vi "ScaledWaveform-GetChannelsRefs.vi"(8 "Error in":errorcluster, 9 "Enabled?":bool, 11 "Device Ref in":T1 format="%.0x") -> (0 "Error out":errorcluster, 2 "Group Data Array":T2(array[cluster]) {"VS Refs" format="%.0x"}, 3 "Device Ref out":T1=18446744073709551615 format="%.0x")   [LabVIEW 2020, in "Waveform-Processing-Custom-Device Shared.lvlib" / "Scaled Waveform.lvlib"]
uses:
  Scaled Waveform.lvlib
  <vilib>/NI VeriStand/Custom Device API/Custom Device Item Ref.ctl
  Constants.vi
  <vilib>/NI VeriStand/Custom Device Tools/Custom Device Utility Library/NI VeriStand - Search for Item by GUID.vi
  <vilib>/NI VeriStand/Custom Device API/Get Item Property (Dependent Node Pointer).vi
  <vilib>/NI VeriStand/Custom Device API/Custom Device API.lvlib
  Waveform-Processing-Custom-Device Shared.lvlib
  <vilib>/NI VeriStand/Custom Device Tools/Custom Device Utility Library/Custom Device Utility Library.lvlib
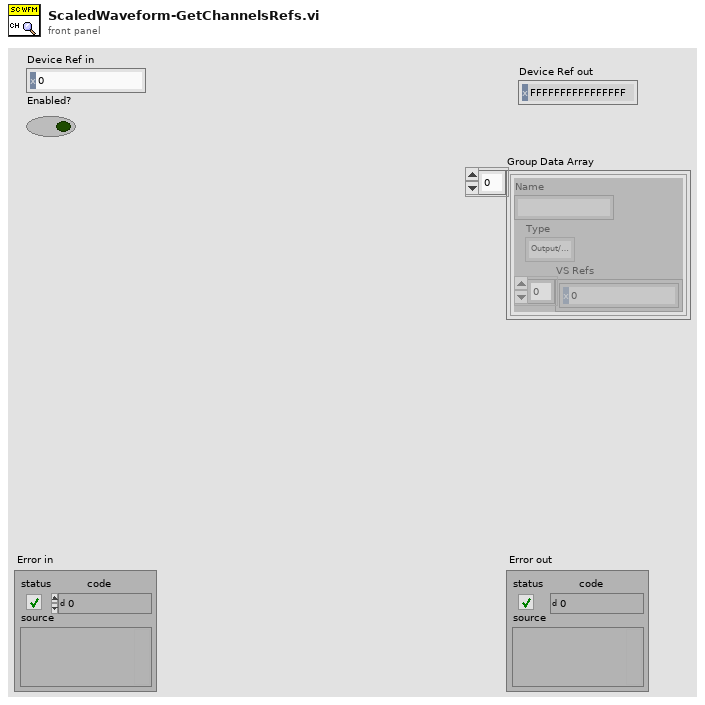
[diagram p1: front panel]
types:
  T1 = typedef "Custom Device API.lvlib/Custom Device Item Ref.ctl" = u64
  T2 = cluster{"Name":string, "Type":enum16{"Output/Write", "Input/Read", "Input/ReadWrite"}, "VS Refs":T1[]}[]
  T3 = enum16{"Output/Write", "Input/Read", "Input/ReadWrite"}
  T4 = cluster{"Name":string, "Type":enum16{"Output/Write", "Input/Read", "Input/ReadWrite"}, "VS Refs":T1[]}
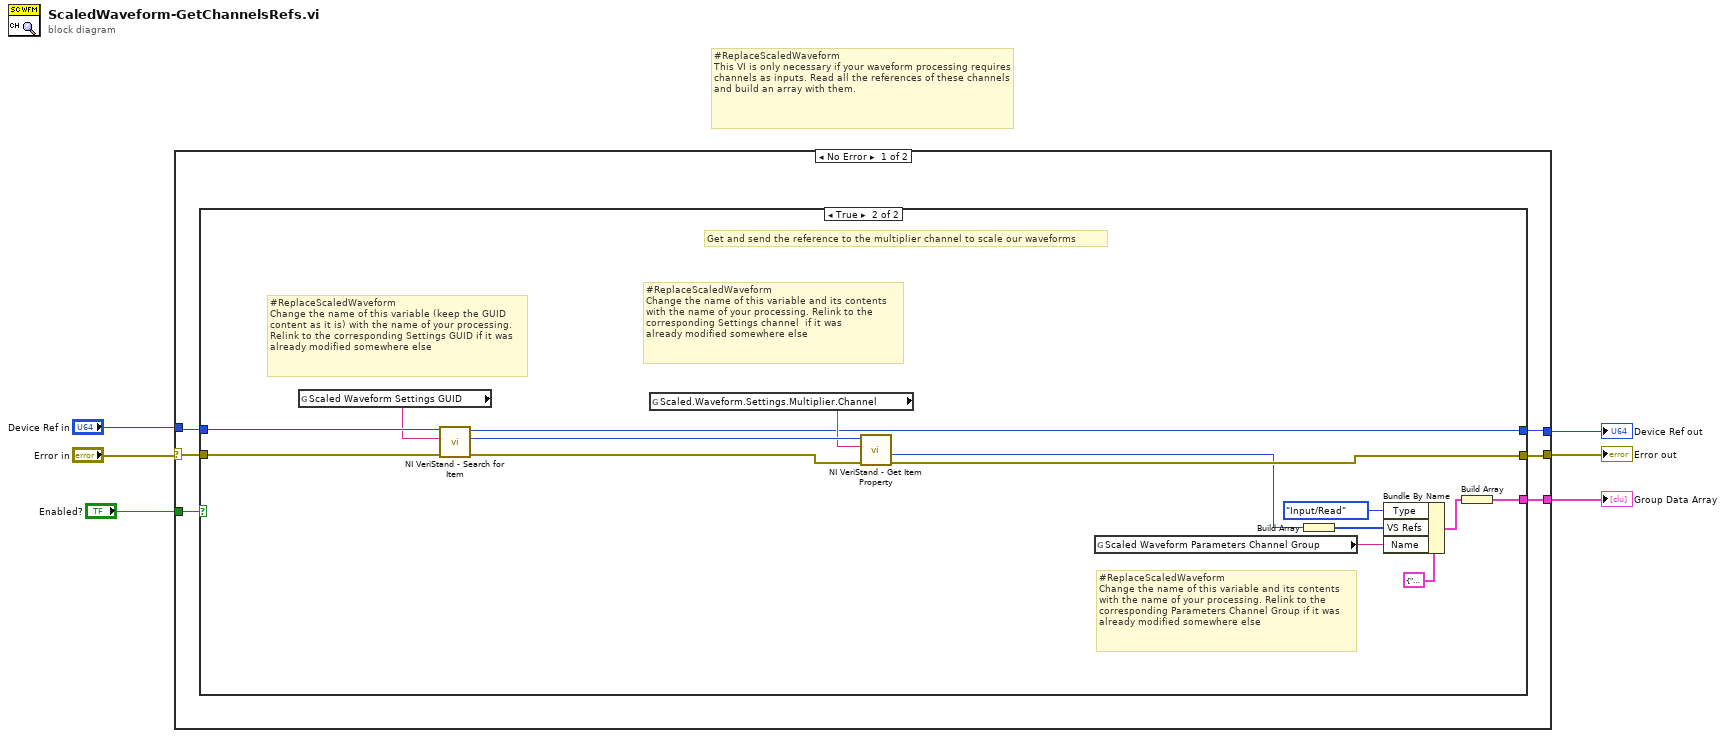
[diagram p0: block diagram]
diagram:
  # "#ReplaceScaledWaveform \nThis VI is only necessary if your waveform processing requires channels as inputs. Read all the references of these channels and build an array with them."
  n1 = case shown="No Error" "Error in" {
    selector: "Error in" -> [w12 w31]
    tunnel: [w10 w31] -> w5
    tunnel: "Device Ref in" -> [w11 w30]
    tunnel: "Enabled?" -> [w9 _]
    tunnel: [w8 w30] -> w2
    tunnel: [w7 _] -> w1
    frame No Error {
      n2 = case shown="True" w9 {
        tunnel: w12 -> [w14 w29]
        tunnel: w11 -> [w13 w28]
        tunnel: [w14 w23] -> w10
        tunnel: [w13 w22] -> w8
        tunnel: [_ w15] -> w7
        frame False {
        }
        frame True {
          # "#ReplaceScaledWaveform \nChange the name of this variable and its contents\nwith the name of your processing. Relink to the\ncorresponding Settings channel  if it was\nalready modified somewhere else"
          # "#ReplaceScaledWaveform \nChange the name of this variable (keep the GUID content as it is) with the name of your processing. Relink to the corresponding Settings GUID if it was\nalready modified somewhere else"
          # "#ReplaceScaledWaveform \nChange the name of this variable and its contents\nwith the name of your processing. Relink to the\ncorresponding Parameters Channel Group if it was\nalready modified somewhere else"
          # "Get and send the reference to the multiplier channel to scale our waveforms"
          n3 = global read "Constants.vi" "Scaled Waveform Settings GUID"() -> (w27:string)
          n4 = call-poly <vilib>:"NI VeriStand - Search for Item.vi"("error in"=w29, "Item GUID"=w27, "Section Ref in"=w28) -> ("error out"=w26:errorcluster, "Item Ref"=w25:T1, "Section Ref out"=w22:T1)  [unwired: 5 in, 1 out]
          n5 = global read "Constants.vi" "Scaled.Waveform.Settings.Multiplier.Channel"() -> (w24:string)
          n6 = call-poly <vilib>:"NI VeriStand - Get Item Property.vi"("error in (no error)"=w26, "Property Name"=w24, "Item Ref in"=w25) -> ("error out"=w23:errorcluster, "Dependent Node Ref"=w18:T1)  [unwired: 5 in, 2 out]
          n7 = global read "Constants.vi" "Scaled Waveform Parameters Channel Group"() -> (w19:string)
          n8 = Build Array(w18) -> (w17:T1[])
          n9 = Bundle By Name(cluster=T4 {"Name"="", "Type"=enum."Output/Write", "VS Refs"=[]} ("Group"), "Type"=T3."Input/Read", "VS Refs"=w17, "Name"=w19) -> (w16:T4)
          n10 = Build Array(w16) -> (w15:T2)
        }
      }
    }
    frame Error {
    }
  }
  "Error out" <- w5
  "Device Ref out" <- w2
  "Group Data Array" <- w1
